vi "Get Completed.vi"(11 "Game in":refnum<class "Game.lvclass">) -> (2 "Completed":bool)   [LabVIEW 2020, in "Conditum-Example.lvlib" / "Game.lvclass"]
uses:
  Game.lvclass
  Conditum/Columns/Boolean/Boolean.lvclass
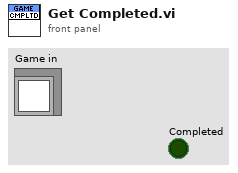
[diagram p1: front panel]
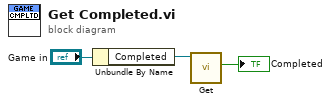
[diagram p0: block diagram]
diagram:
  n1 = Unbundle By Name("Game in") -> ("Completed"=w2:refnum<class "Boolean.lvclass">)
  n2 = call "Get.vi"("Boolean in"=w2) -> ("Value"=→"Completed":bool)  [unwired: 10 in]
